vi "temperature_controller.vi"() -> ()   [LabVIEW 2017]
panel:
  out "?":u32
  in  "time interval to wait":dbl
  in  "Temo diff":dbl
  out "return count":u32
  in  "VISA resource name":refnum<visa-resource-name>
  in  "End Temp":dbl
  in  "Start Temp":dbl
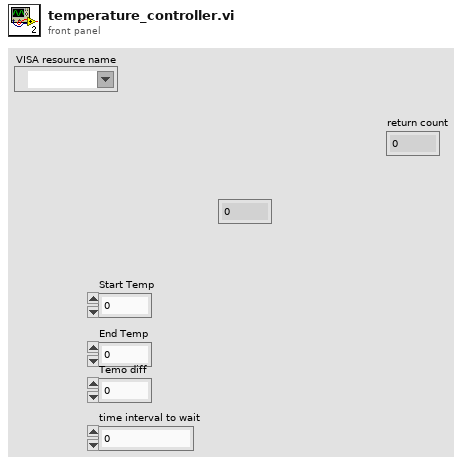
[diagram p1: front panel]
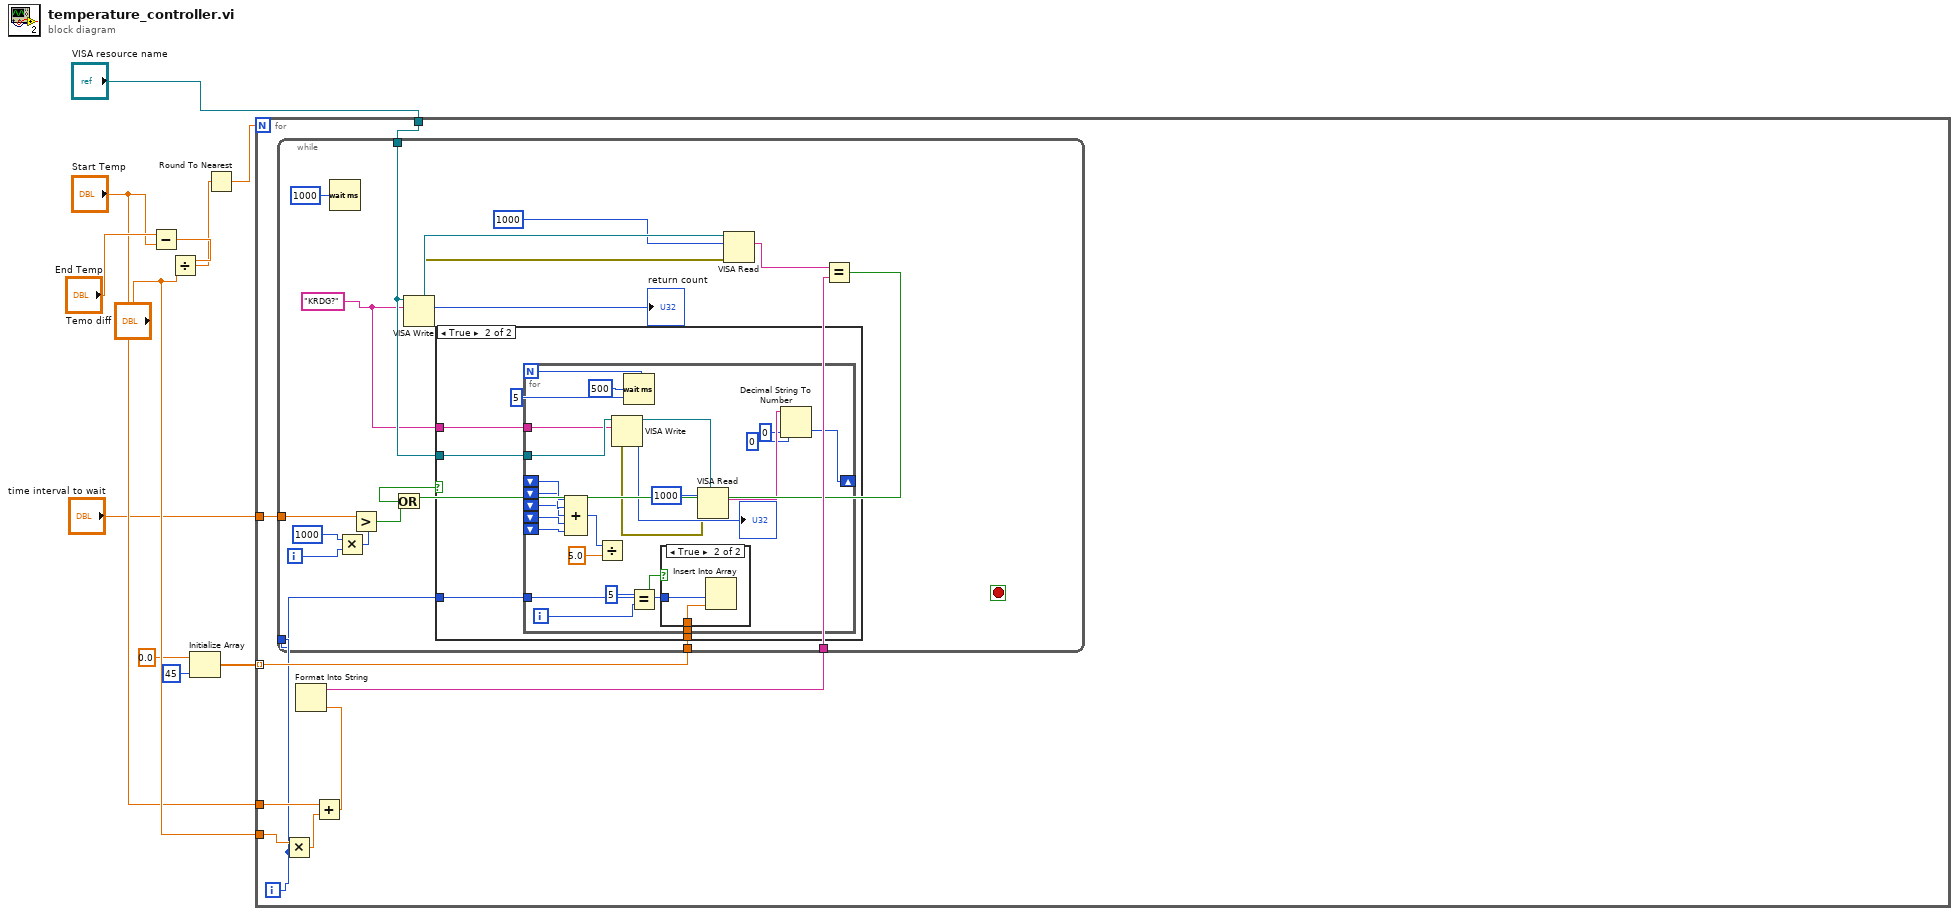
[diagram p0: block diagram]
diagram:
  n1 = Subtract(x="End Temp", y="Start Temp") -> (x-y=w10:dbl)
  n2 = Divide(x=w10, y="Temo diff") -> (x/y=w9:dbl)
  n3 = Initialize Array(0.0 ("element"), 45 ("dimension size")) -> (w2:dbl[])
  n4 = Round To Nearest(number=w9) -> (nearest integer value=w8:dbl)
  n5 = for {
    N: w8 -> [_]
    tunnel: "Temo diff" -> [w20]
    tunnel: "Start Temp" -> [w19]
    tunnel: "VISA resource name" -> [w16]
    tunnel: "time interval to wait" -> [w14]
    tunnel: w2 -> [w13] mode=indexing
    i -> [w12]
    n6 = Multiply(x=w20, y=w12) -> (x*y=w18:dbl)
    n7 = Add(x=w19, y=w18) -> (x+y=w17:dbl)
    n8 = Format Into String(w17) -> (resulting string=w15:string)  [unwired: 3 in, 1 out]
    n9 = while {
      tunnel: w16 -> [w27]
      tunnel: w15 -> [w33]
      tunnel: w14 -> [w28]
      tunnel: w13 -> [w26]
      tunnel: w12 -> [w21]
      i -> [w31]
      stop <- _ stop-if-true
      w22 = "KRDG?" ("write buffer")
      n10 = Wait (ms)(milliseconds to wait=u32 1000) -> ()  [unwired: 1 out]
      n11 = Multiply(x=1000, y=w31) -> (x*y=w29:i32)
      n12 = Greater?(x=w28, y=w29) -> (0:w25:bool)
      n13 = VISA Write(VISA resource name=w27, write buffer=w22) -> (VISA resource name out=w37:refnum<visa-resource-name>, return count=→"return count":u32, error out=w35:errorcluster)  [unwired: 1 in]
      n14 = VISA Read(VISA resource name=w37, byte count=u32 1000, error in (no error)=w35) -> (read buffer=w32:string)  [unwired: 3 out]
      n15 = Equal?(x=w32, y=w33) -> (x = y?=w23:bool)
      n16 = Or(x=w23, y=w25) -> (x .or. y?=w24:bool)
      n17 = case shown="True" w24 {
        tunnel: w27 -> [_ w42]
        tunnel: w26 -> [_ w41]
        tunnel: w22 -> [_ w40]
        tunnel: w21 -> [_ w39]
        frame False {
        }
        frame True {
          n18 = for {
            N: 5 -> [_]
            tunnel: w42 -> [w63]
            shift-right: [w57] -> _
            shift-left: _ -> [w56]
            shift-left: _ -> [w55]
            shift-left: _ -> [w54]
            shift-left: _ -> [w53]
            shift-left: _ -> [w52]
            tunnel: w41 -> [w46]
            tunnel: w40 -> [w45]
            tunnel: w39 -> [w44]
            i -> [w49]
            n19 = Compound Arithmetic op=ADD(w56, w55, w54, w53, w52) -> (w50:i32)
            n20 = Divide(x=w50, y=5.0) -> ()  [unwired: 1 out]
            n21 = VISA Write(VISA resource name=w63, write buffer=w45) -> (VISA resource name out=w62:refnum<visa-resource-name>, return count=→"?":u32, error out=w65:errorcluster)  [unwired: 1 in]
            n22 = Wait (ms)(milliseconds to wait=u32 500) -> ()  [unwired: 1 out]
            n23 = Equal?(x=5, y=w49) -> (x = y?=w47:bool)
            n24 = case shown="True" w47 {
              tunnel: w46 -> [_ w68]
              tunnel: w44 -> [_ w67]
              frame False {
              }
              frame True {
                n25 = Insert Into Array(index=w67, new element=w68) -> ()  [unwired: 1 in, 1 out]
              }
            }
            n26 = VISA Read(VISA resource name=w62, byte count=u32 1000, error in (no error)=w65) -> (read buffer=w60:string)  [unwired: 3 out]
            n27 = Decimal String To Number(string=w60, offset=0, default (0L)=0 ("default (0 I32)")) -> (number=w57:i32)  [unwired: 1 out]
          }
        }
      }
    }
  }
